vi "170731-BM.vi"() -> ()   [LabVIEW 2017]
uses:
  Global_InitEndSync.vi
panel:
  in  "nVista":bool
  in  "noise":bool
  out "Elapsed Time Text":string caption="Start Time Text"
  out "error out 2":errorcluster
  out "error out":errorcluster
  in  "Top Button":bool
  in  "Gate Close / END Button":bool
  in  "Start Button":bool
  in  "ID":u8=1 min=1 step=1
  in  "Trial":u8=1 min=1 max=3 step=1
  in  "Phase":enum32{"Habituation", "Training", "Probe test"}(radio)=enum."Training"
  in  "Entry":enum8{"Lift", "Start-box", "Manual"}(ring)
  out "Mem usage (%)*":u8(slide) caption="Slide 2" scale=0.0..100.0
  out "Save Path":path
  in  "Day":u8 max=20 step=1
  in  "Project Path":path
  in  "Frequency (Hz)":dbl=20.0
  out "General State":string
  # "*Restart the program, if the memory usage exceeded 70%."
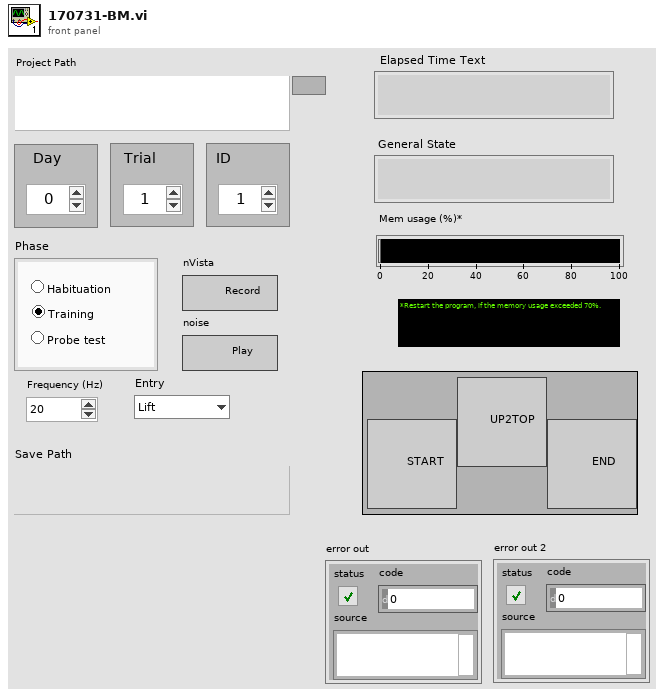
[diagram p1: front panel]
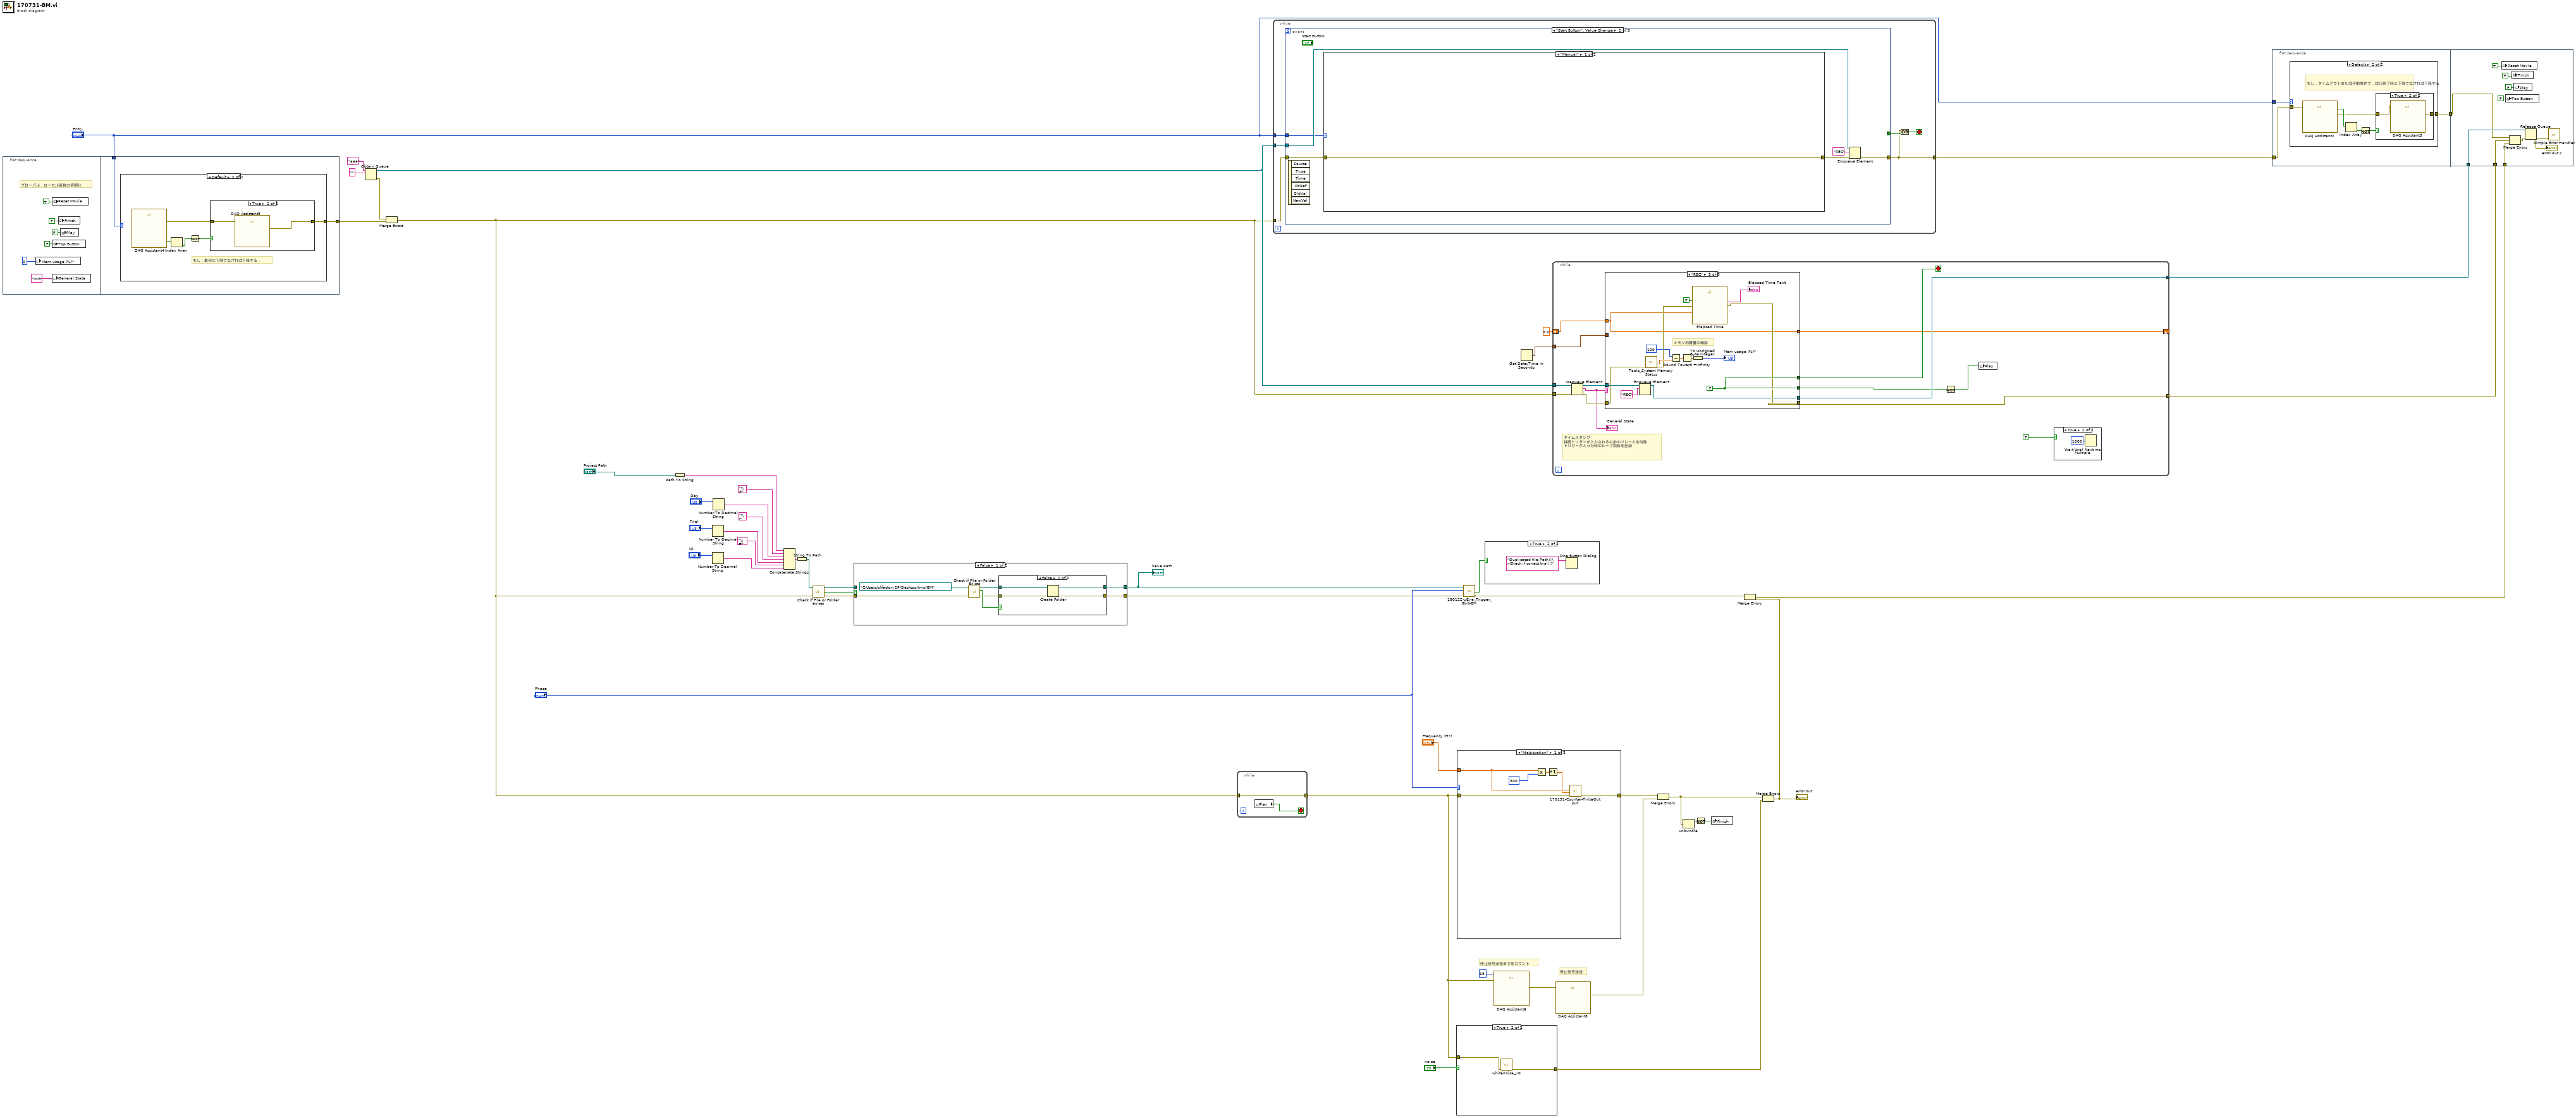
[diagram p0: block diagram]
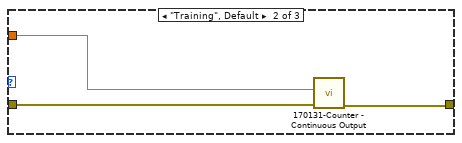
[diagram p4: hidden frame]
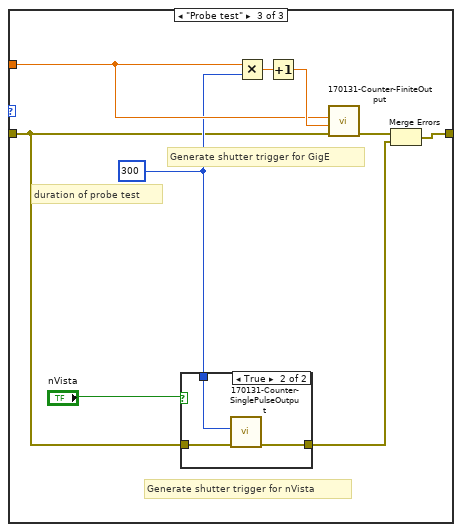
[diagram p5: hidden frame]
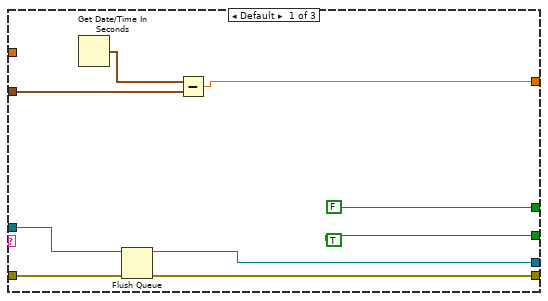
[diagram p10: hidden frame]
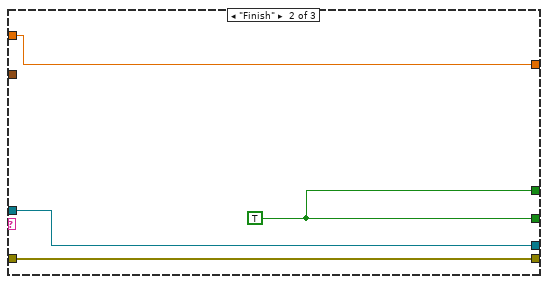
[diagram p11: hidden frame]
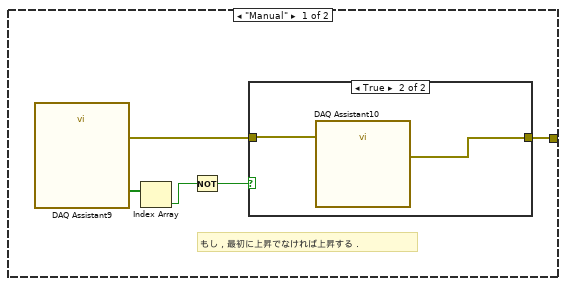
[diagram p12: hidden frame]
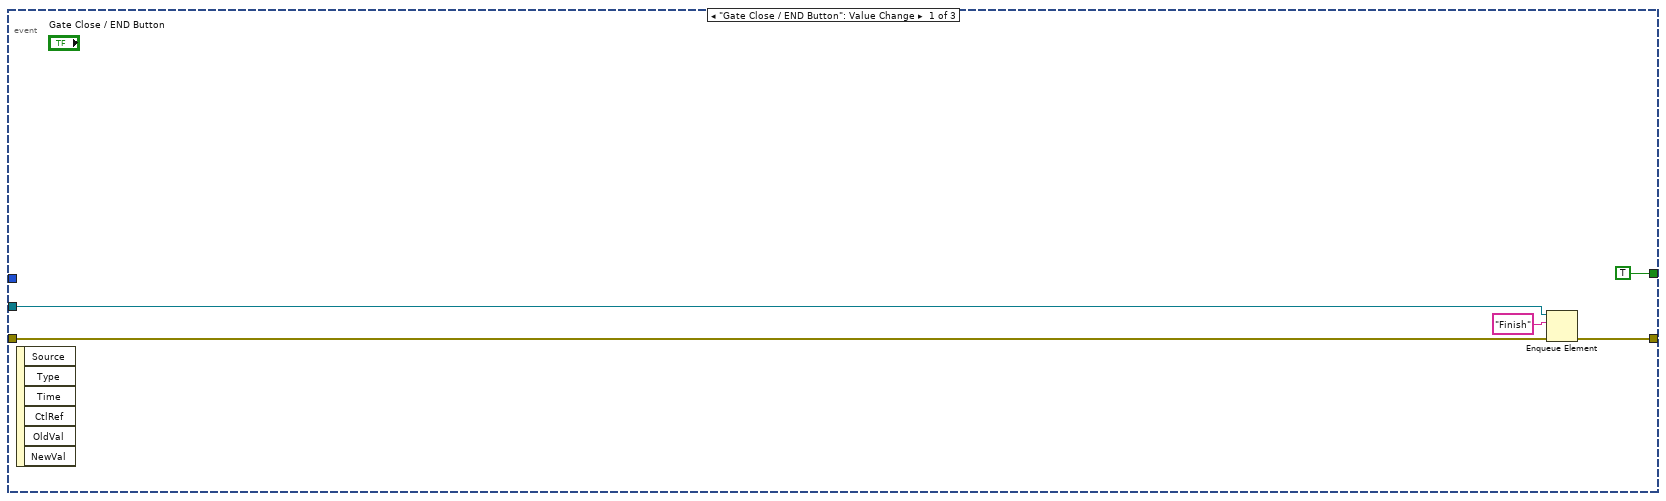
[diagram p17: hidden frame]
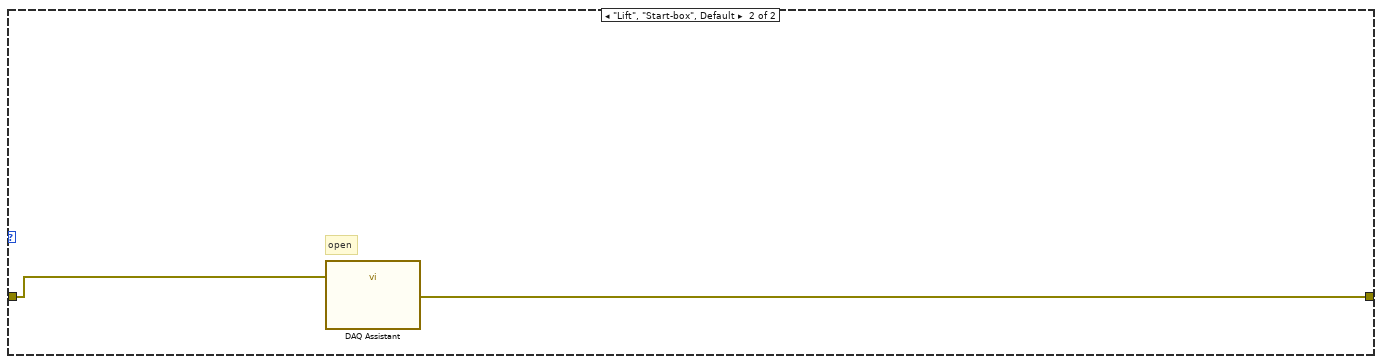
[diagram p18: hidden frame]
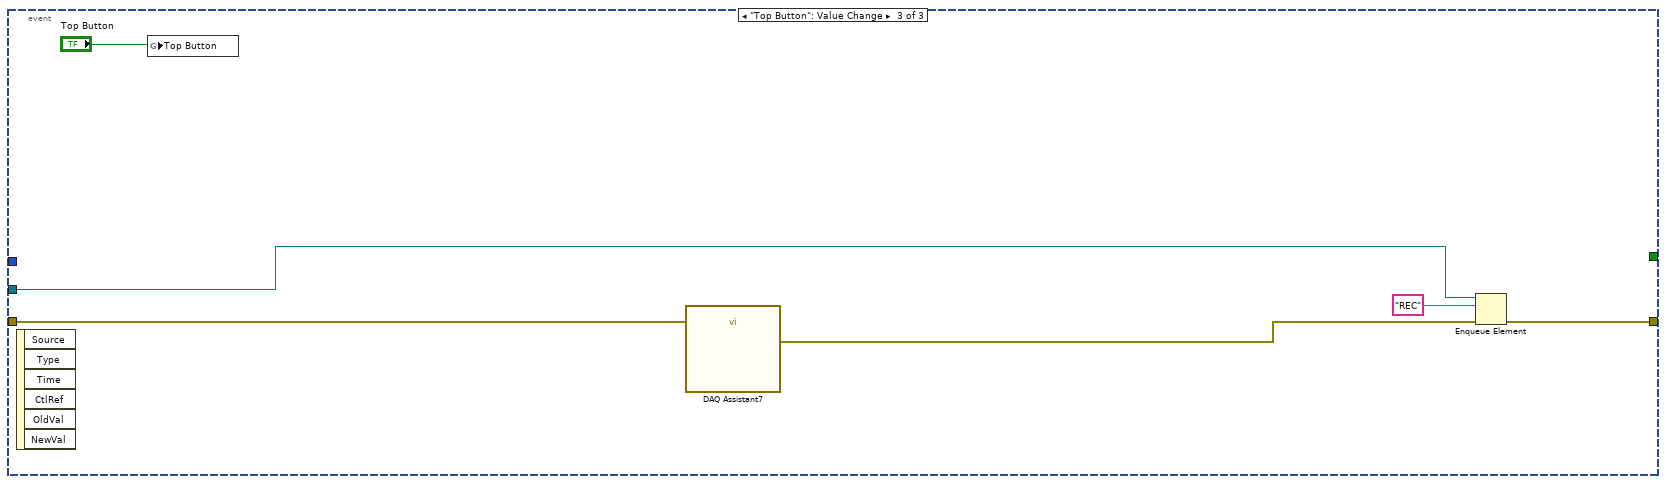
[diagram p19: hidden frame]
diagram:
  # "停止信号送信"
  # "停止信号送信までをカウント"
  n1 = flat-sequence {
    tunnel: [w55] -> w42
    tunnel: "Entry" -> [w54]
    frame #0 {
      # "グローバル，ローカル変数の初期化"
      n2 = local write "Mem usage (%)*"(0) -> ()
      n3 = global write "Global_InitEndSync.vi" "Top Button"(FALSE ("Top Button")) -> ()
      n4 = global write "Global_InitEndSync.vi" "Reset Movie"(TRUE) -> ()
      n5 = local write "General State"("Init") -> ()
      n6 = global write "Global_InitEndSync.vi" "Finish"(FALSE) -> ()
      n7 = global write "Global_InitEndSync.vi" "Play"(FALSE ("Play")) -> ()
    }
    frame #1 {
      n8 = case shown="Default" w54 {
        tunnel: [w56 w65] -> w55
        frame "Manual" {
          # "もし，最初に上昇でなければ上昇する．"
          n9 = call "DAQ Assistant9"() -> ("data"=w60:bool[], "error out"=w58:errorcluster)  [unwired: 17 in, 1 out]
          n10 = Index Array(array=w60) -> (element=w59:bool)  [unwired: 1 in]
          n11 = Not(x=w59) -> (.not. x?=w57:bool)
          n12 = case shown="True" w57 {
            tunnel: [w61 w63] -> w56
            tunnel: w58 -> [w61 w62]
            frame False {
            }
            frame True {
              n13 = call "DAQ Assistant10"("error in"=w62) -> ("error out"=w63:errorcluster)  [unwired: 17 in, 1 out]
            }
          }
        }
        frame Default {
          # "もし，最初に下降でなければ下降する．"
          n14 = call "DAQ Assistant4"() -> ("data"=w68:bool[], "error out"=w66:errorcluster)  [unwired: 17 in, 1 out]
          n15 = Index Array(array=w68) -> (element=w67:bool)  [unwired: 1 in]
          n16 = Not(x=w67) -> (.not. x?=w64:bool)
          n17 = case shown="True" w64 {
            tunnel: [w69 w71] -> w65
            tunnel: w66 -> [w69 w70]
            frame False {
            }
            frame True {
              n18 = call "DAQ Assistant5"("error in"=w70) -> ("error out"=w71:errorcluster)  [unwired: 17 in, 1 out]
            }
          }
        }
      }
    }
  }
  n19 = Obtain Queue(name (unnamed)="aaa", element data type="" ("element")) -> (queue out=w43:refnum<queue>, error out=w46:errorcluster)  [unwired: 3 in, 1 out]
  n20 = Merge Errors(w46, w42) -> (w23:errorcluster)
  n21 = Path To String(path="Project Path") -> (string=w17:string)
  n22 = Number To Decimal String(number="ID") -> (decimal integer string=w29:string)  [unwired: 1 in]
  n23 = Number To Decimal String(number="Trial") -> (decimal integer string=w31:string)  [unwired: 1 in]
  n24 = Number To Decimal String(number="Day") -> (decimal integer string=w34:string)  [unwired: 1 in]
  n25 = Concatenate Strings(w17, "\\d", w34, "\\t", w31, "\\#", w29) -> (w27:string)
  n26 = String To Path(string=w27) -> (path=w28:path)
  n27 = call <vilib>:"Check if File or Folder Exists.vi"("error in (no error)"=w23, "path"=w28) -> ("error out"=w24:errorcluster, "file or folder exists?"=w25:bool, "dup path"=w26:path)  [unwired: 7 in]
  n28 = case shown="False" w25 {
    tunnel: [w78 w86] -> w14
    tunnel: w26 -> [_ w86]
    tunnel: w24 -> [w76 w85]
    tunnel: [w72 w85] -> w12
    frame False {
      n29 = call <vilib>:"Check if File or Folder Exists.vi"("error in (no error)"=w76, "path"=path "C:/Users/olfactory2P/Desktop/tmp/BM" ("dup path")) -> ("error out"=w73:errorcluster, "file or folder exists?"=w75:bool, "dup path"=w74:path)  [unwired: 7 in]
      n30 = case shown="False" w75 {
        tunnel: [w82 w84] -> w78
        tunnel: w74 -> [w81 w84]
        tunnel: w73 -> [w80 w83]
        tunnel: [w79 w83] -> w72
        frame False {
          n31 = Create Folder(path (use dialog)=w81, error in=w80) -> (created path=w82:path, error out=w79:errorcluster)  [unwired: 1 in, 1 out]
        }
        frame True {
        }
      }
    }
    frame True {
    }
  }
  "Save Path" <- w14
  n32 = while {
    tunnel: w23 -> [w88]
    tunnel: [w88] -> w3
    stop <- w87 stop-if-true
    n33 = global read "Global_InitEndSync.vi" "Play"() -> (w87:bool)
  }
  n34 = while {
    tunnel: [w91] -> w47
    tunnel: w23 -> [w93]
    tunnel: w43 -> [w90]
    tunnel: "Entry" -> [w89]
    stop <- w92 stop-if-true
    n35 = event shown="[1] \"Start Button\": Value Change" {
      selector: _ -> [_ _ _]
      dyn-events: _ -> [_ _ _]
      timeout: _ -> [_ _ _]
      tunnel: [TRUE _ _] -> w94
      tunnel: [w96 w104 w112] -> w91
      tunnel: w93 -> [w97 w102 w110]
      tunnel: w90 -> [w98 w105 w113]
      tunnel: w89 -> [_ w100 _]
      event "Gate Close / END Button": Value Change {
        n36 = event-data() -> ()  [unwired: 1 in, 6 out]
        n37 = Enqueue Element(queue=w98, element="Finish", error in (no error)=w97) -> (error out=w96:errorcluster)  [unwired: 1 in, 2 out]
      }
      event "Start Button": Value Change {
        n38 = event-data() -> ()  [unwired: 1 in, 6 out]
        n39 = case shown="\"Manual\"" w100 {
          tunnel: w102 -> [w106 w107]
          tunnel: [w106 w108] -> w101
          frame "Manual" {
          }
          frame "Lift", "Start-box", Default {
            # "open"
            n40 = call "DAQ Assistant"("error in"=w107) -> ("error out"=w108:errorcluster)  [unwired: 17 in, 1 out]
          }
        }
        n41 = Enqueue Element(queue=w105, element="REC", error in (no error)=w101) -> (error out=w104:errorcluster)  [unwired: 1 in, 2 out]
      }
      event "Top Button": Value Change {
        n42 = event-data() -> ()  [unwired: 1 in, 6 out]
        n43 = global write "Global_InitEndSync.vi" "Top Button"("Top Button") -> ()
        n44 = call "DAQ Assistant7"("error in"=w110) -> ("error out"=w111:errorcluster)  [unwired: 17 in, 1 out]
        n45 = Enqueue Element(queue=w113, element="REC", error in (no error)=w111) -> (error out=w112:errorcluster)  [unwired: 1 in, 2 out]
      }
    }
    n46 = Or(x=w91, y=w94) -> (x .or. y?=w92:bool)
  }
  n47 = case shown="True" "noise" {
    tunnel: w3 -> [w115 w116]
    tunnel: [w115 w117] -> w1
    frame False {
    }
    frame True {
      n48 = call "whitenoise_v0.vi"("error in (no error)"=w116) -> ("error out"=w117:errorcluster)  [unwired: 10 in]
    }
  }
  n49 = case shown="\"Habituation\"" "Phase" {
    tunnel: w3 -> [w123 w125 w130]
    tunnel: [w122 w124 w129] -> w19
    tunnel: "Frequency (Hz)" -> [w121 w126 w133]
    frame "Habituation" {
      n50 = Multiply(x=w121, y=300) -> (x*y=w119:dbl)
      n51 = Increment(x=w119) -> (x+1=w120:dbl)
      n52 = call "170131-Counter-FiniteOutput.vi"("error in"=w123, "Number of Pulses"=w120, "Frequency"=w121) -> ("error out 2"=w122:errorcluster)  [unwired: 8 in]
    }
    frame "Training", Default {
      n53 = call "170131-Counter - Continuous Output.vi"("error in"=w125, "Frequency"=w126) -> ("error out 2"=w124:errorcluster)  [unwired: 9 in]
    }
    frame "Probe test" {
      w131 = 300
      # "Generate shutter trigger for nVista"
      # "Generate shutter trigger for GigE"
      # "duration of probe test"
      n54 = case shown="True" "nVista" {
        tunnel: w131 -> [_ w139]
        tunnel: w130 -> [w136 w138]
        tunnel: [w136 w137] -> w128
        frame False {
        }
        frame True {
          n55 = call "170131-Counter-SinglePulseOutput.vi"("error in"=w138, "Pulse Duration"=w139) -> ("error out 2"=w137:errorcluster)  [unwired: 9 in]
        }
      }
      n56 = Multiply(x=w133, y=w131) -> (x*y=w134:dbl)
      n57 = Increment(x=w134) -> (x+1=w135:dbl)
      n58 = call "170131-Counter-FiniteOutput.vi"("error in"=w130, "Number of Pulses"=w135, "Frequency"=w133) -> ("error out 2"=w132:errorcluster)  [unwired: 8 in]
      n59 = Merge Errors(w132, w128) -> (w129:errorcluster)
    }
  }
  n60 = call "180122-uEye_Trigger_8bit-BM.vi"("error in"=w12, "Phase"="Phase", "Save Path"=w14) -> ("error out"=w10:errorcluster, "DupFiles"=w11:bool)  [unwired: 5 in]
  n61 = case shown="True" w11 {
    frame False {
    }
    frame True {
      n62 = One Button Dialog(message="Duplicated file Path!!!\nCheck if correct trial!!!" ("error source (\" \")")) -> ()  [unwired: 1 in, 1 out]
    }
  }
  n63 = call "DAQ Assistant6"("number of samples"=65, "error in"=w3) -> ("error out"=w20:errorcluster)  [unwired: 16 in, 1 out]
  n64 = Get Date/Time In Seconds() -> (seconds since 1Jan1904=w6:timestamp)
  n65 = while {
    tunnel: w43 -> [w154]
    tunnel: [w149] -> w40
    tunnel: w23 -> [w153]
    tunnel: [w146] -> w39
    tunnel: w6 -> [w143]
    shift-right: [w142] -> _
    shift-left: 0.0 -> [w141]
    stop <- w148 stop-if-true
    # "タイムスタンプ\n録画トリガーが入力される以前のフレームを削除\nトリガーが入った時のループ回数を記録"
    n66 = Dequeue Element(queue=w154, error in (no error)=w153) -> (queue out=w151:refnum<queue>, element=w150:string, error out=w152:errorcluster)  [unwired: 1 in, 1 out]
    "General State" <- w150
    n67 = case shown="\"REC\"" w150 {
      tunnel: [TRUE w167 w180] -> w145
      tunnel: w152 -> [w161 w166 w172]
      tunnel: [w160 w166 w171] -> w146
      tunnel: w151 -> [w163 w168 w183]
      tunnel: [w162 w168 w182] -> w149
      tunnel: [FALSE w167 w180] -> w148
      tunnel: w143 -> [w157 _ _]
      tunnel: [w156 w165 w170] -> w142
      tunnel: w141 -> [_ w165 w170]
      frame Default {
        n68 = Get Date/Time In Seconds() -> (seconds since 1Jan1904=w158:timestamp)
        n69 = Flush Queue(queue=w163, error in (no error)=w161) -> (queue out=w162:refnum<queue>, error out=w160:errorcluster)  [unwired: 1 out]
        n70 = Subtract(x=w158, y=w157) -> (x-y=w156:dbl)
      }
      frame "Finish" {
        w167 = TRUE
      }
      frame "REC" {
        w180 = FALSE
        # "メモリ消費量の確認"
        n71 = Enqueue Element(queue=w183, element="REC") -> (queue out=w182:refnum<queue>)  [unwired: 2 in, 2 out]
        n72 = call "Tools_System Memory Status.vi"("error in (no error)"=w172) -> ("error out"=w173:errorcluster, "Free memory (%)"=w175:dbl)  [unwired: 7 in, 2 out]
        n73 = Subtract(x=100, y=w175) -> (x-y=w177:dbl)
        n74 = Round Toward +Infinity(x=w177) -> (ceil(x): smallest int >= x=w178:dbl)
        n75 = To Unsigned Byte Integer(number=w178) -> (unsigned 8bit integer=→"Mem usage (%)*":u8)
        n76 = call "Elapsed Time"("Auto Reset"=FALSE, "error in (no error)"=w173, "Set Start Time (s)"=w170) -> ("Elapsed Time Text"=→"Elapsed Time Text":string, "error out"=w171:errorcluster)  [unwired: 9 in, 6 out]
      }
    }
    n77 = Not(x=w145) -> (.not. x?=w144:bool)
    n78 = global write "Global_InitEndSync.vi" "Play"(w144) -> ()
    n79 = case shown="True" TRUE {
      frame False {
      }
      frame True {
        n80 = Wait Until Next ms Multiple(millisecond multiple=u32 1000) -> ()  [unwired: 1 out]
      }
    }
  }
  n81 = call "DAQ Assistant8"("error in"=w20) -> ("error out"=w18:errorcluster)  [unwired: 17 in, 1 out]
  n82 = Merge Errors(w19, w18) -> (w9:errorcluster)
  n83 = Unbundle(w9) -> ("status"=w8:bool)  [unwired: 2 out]
  n84 = Not(x=w8) -> (.not. x?=w7:bool)
  n85 = global write "Global_InitEndSync.vi" "Finish"(w7) -> ()
  n86 = Merge Errors(w9, w1) -> (w2:errorcluster)
  "error out" <- w2
  n87 = Merge Errors(w10, w2) -> (w38:errorcluster)
  n88 = flat-sequence {
    tunnel: w47 -> [w184]
    tunnel: [w186] -> w41
    tunnel: "Entry" -> [w185]
    tunnel: w41 -> [w197]
    tunnel: w40 -> [w205]
    tunnel: w39 -> [w203]
    tunnel: w38 -> [w204]
    frame #0 {
      n89 = case shown="Default" w185 {
        tunnel: [w187 w193] -> w186
        tunnel: w184 -> [w187 w188]
        frame "Manual" {
        }
        frame Default {
          # "もし，タイムアウトまたは手動操作で，試行終了時に下降でなければ下降する"
          n90 = call "DAQ Assistant2"("error in"=w188) -> ("data"=w192:bool[], "error out"=w191:errorcluster)  [unwired: 16 in, 1 out]
          n91 = Index Array(array=w192) -> (element=w190:bool)  [unwired: 1 in]
          n92 = Not(x=w190) -> (.not. x?=w189:bool)
          n93 = case shown="True" w189 {
            tunnel: [w194 w196] -> w193
            tunnel: w191 -> [w194 w195]
            frame False {
            }
            frame True {
              n94 = call "DAQ Assistant3"("error in"=w195) -> ("error out"=w196:errorcluster)  [unwired: 17 in, 1 out]
            }
          }
        }
      }
    }
    frame #1 {
      n95 = global write "Global_InitEndSync.vi" "Reset Movie"(TRUE) -> ()
      n96 = global write "Global_InitEndSync.vi" "Top Button"(FALSE ("Top Button")) -> ()
      n97 = Merge Errors(w197, w203, w204) -> (w206:errorcluster)
      n98 = global write "Global_InitEndSync.vi" "Finish"(FALSE) -> ()
      n99 = global write "Global_InitEndSync.vi" "Play"(FALSE ("Play")) -> ()
      n100 = Release Queue(queue=w205, error in (no error)=w206) -> (error out=w202:errorcluster)  [unwired: 1 in, 2 out]
      "error out 2" <- w202
      n101 = call <vilib>:"Simple Error Handler.vi"("error in (no error)"=w202) -> ()  [unwired: 4 in, 5 out]
    }
  }
